vi "Get Process ID from Monkey.vi"(8 "error in (no error)":errorcluster, 10 "Monkey ID":string, 11 "Tamer in":refnum<class "Tamer.lvclass">) -> (0 "error out":errorcluster, 2 "Process ID":string, 3 "Tamer out":refnum<class "Tamer.lvclass">)   [LabVIEW 2020, in "CIRCUS_uServices.lvlib" / "Tamer.lvlib" / "Tamer.lvclass"]
uses:
  Tamer.lvclass
  Tamer.lvclass/Tamer.ctl
  TALOS/TALOS_PPL.lvlibp
  C:/Users/marco/Documents/GitHub_Lab/CIRCUS/TALOS/TALOS_PPL.lvlibp/Father of all uServices/Father of all uServices/Father of all uServices.lvclass
  C:/Users/marco/Documents/GitHub_Lab/CIRCUS/TALOS/TALOS_PPL.lvlibp/Ancestor/Ancestor/Ancestor.lvclass
  C:/Users/marco/Documents/GitHub_Lab/CIRCUS/TALOS/Actor Framework.lvlibp/1abvi3w/vi.lib/ActorFramework/Actor/Actor.lvclass
  C:/Users/marco/Documents/GitHub_Lab/CIRCUS/CIRCUS uServices et al/Tamer/Tamer.lvclass
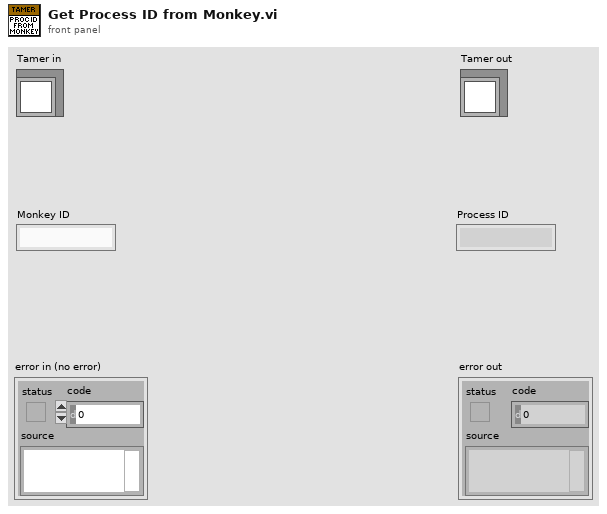
[diagram p1: front panel]
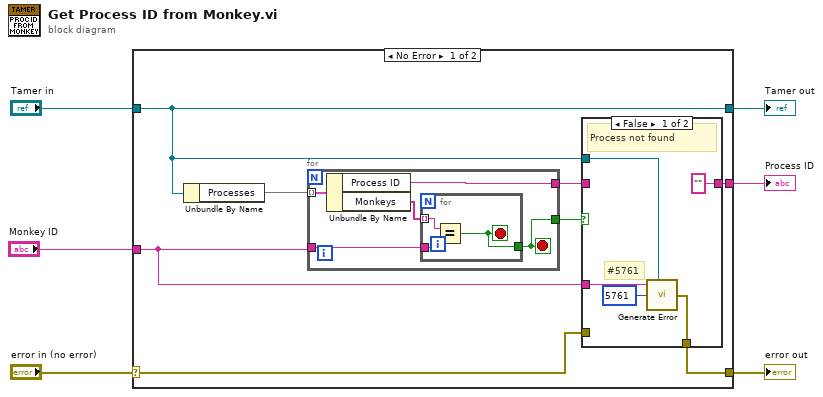
[diagram p0: block diagram]
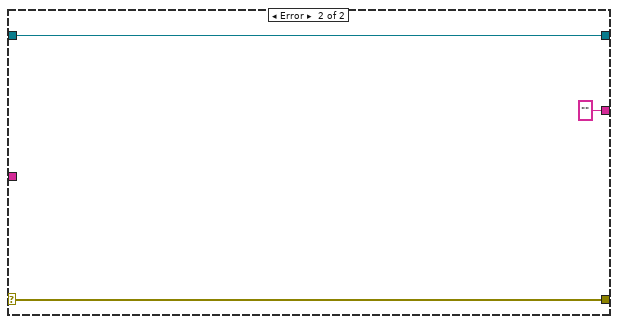
[diagram p3: hidden frame]
diagram:
  n1 = case shown="No Error" "error in (no error)" {
    selector: "error in (no error)" -> [w8 w32]
    tunnel: [w9 w32] -> w5
    tunnel: [w10 w31] -> w3
    tunnel: "Tamer in" -> [w10 w31]
    tunnel: "Monkey ID" -> [w7 _]
    tunnel: [w11 "" ("Process ID")] -> w1
    frame No Error {
      n2 = Unbundle By Name(w10) -> ("Processes"=w14:map{string, string[]})
      n3 = for {
        tunnel: w14 -> [w26] mode=indexing
        tunnel: w7 -> [w24]
        tunnel: [w23] -> w12
        tunnel: [w22] -> w13
        stop <- w22 stop-if-true
        n4 = Unbundle By Name(w26) -> ("Process ID"=w23:string, "Monkeys"=w25:string[])
        n5 = for {
          tunnel: w25 -> [w29] mode=indexing
          tunnel: w24 -> [w28]
          tunnel: [w27] -> w22
          stop <- w27 stop-if-true
          n6 = Equal?(x=w29, y=w28) -> (x = y?=w27:bool)
        }
      }
      n7 = case shown="False" w13 {
        tunnel: w12 -> [_ w21]
        tunnel: ["" ("Process ID") w21] -> w11
        tunnel: w10 -> [w18 _]
        tunnel: [w17 w20] -> w9
        tunnel: w8 -> [_ w20]
        tunnel: w7 -> [w16 _]
        frame False {
          # "#5761"
          # "Process not found"
          n8 = call "Generate Error.vi"("Optional String"=w16, "Class"=w18, "Error Code"=5761) -> ("error out"=w17:errorcluster)  [unwired: 4 in]
        }
        frame True {
          # "Process found"
        }
      }
    }
    frame Error {
    }
  }
  "error out" <- w5
  "Tamer out" <- w3
  "Process ID" <- w1
